vi "ConfigUtilities - Packet Tx or Rx.vi"(8 "error in (no error)":errorcluster, 11 "Item Ref in":T1 format="%.0x") -> (0 "error out":errorcluster, 2 "Tx?":bool, 3 "Item Ref out":T1 format="%.0x")   [LabVIEW 2015, in "UDP-Custom-Device System Explorer.lvlib"]
uses:
  UDP-Custom-Device System Explorer.lvlib
  <vilib>/NI Veristand/Custom Device API/Custom Device Item Ref.ctl
  <vilib>/NI VeriStand/Custom Device API/Custom Device API.lvlib
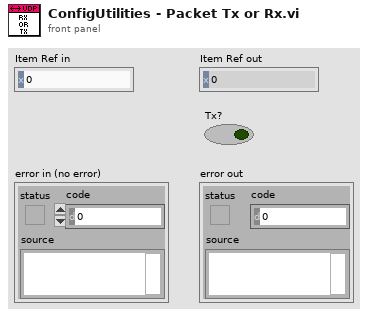
[diagram p1: front panel]
types:
  T1 = typedef "Custom Device API.lvlib/Custom Device Item Ref.ctl" = u64
  T2 = typedef "Custom Device API.lvlib/Custom Device Item Info.ctl" = cluster{"Name":string, "Is Channel":bool, "GUID":string, "Is Waveform":bool}
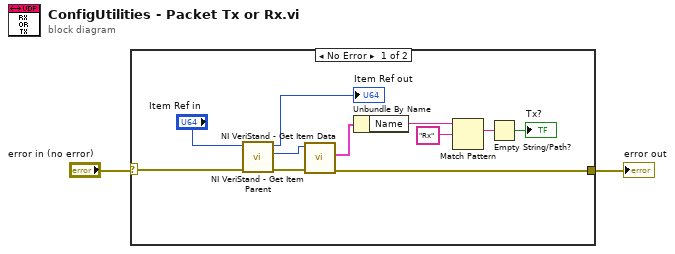
[diagram p0: block diagram]
diagram:
  n1 = case shown="No Error" "error in (no error)" {
    selector: "error in (no error)" -> [w9 w14]
    tunnel: [w10 w14] -> w2
    frame No Error {
      n2 = call <vilib>:"NI VeriStand - Get Item Parent.vi"("error in (no error)"=w9, "Item Ref in"="Item Ref in") -> ("error out"=w6:errorcluster, "Parent Ref"=w3:T1, "Item Ref out"=→"Item Ref out":T1)  [unwired: 6 in, 1 out]
      n3 = call <vilib>:"NI VeriStand - Get Item Data.vi"("error in (no error)"=w6, "Item Ref in"=w3) -> ("error out"=w10:errorcluster, "Item Info"=w11:T2)  [unwired: 6 in, 2 out]
      n4 = Unbundle By Name(w11) -> ("Name"=w8:string)
      n5 = Match Pattern(string=w8, regular expression="Rx") -> (match substring=w7:string)  [unwired: 1 in, 3 out]
      n6 = Empty String/Path?(string/path=w7) -> (empty?=→"Tx?":bool)
    }
    frame Error {
    }
  }
  "error out" <- w2
